vi "CVT_FGV.vi"(0 "command":enum16{"set", "get", "reset", "get all"}(ring), 5 "variable":string, 7 "value in":string, 9 "compressed":bool, 11 "error in":errorcluster) -> (4 "value out":string, 6 "all out":variant, 15 "error out":errorcluster)   [LabVIEW 2011]
panel:
  out "uncompressed":variant
  out "compressed":variant
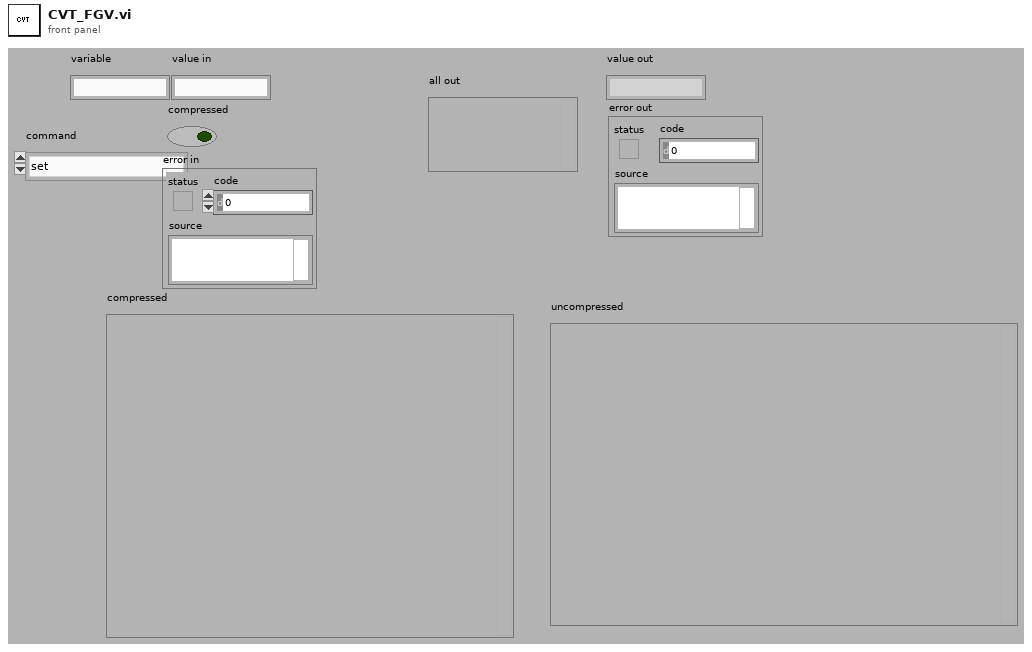
[diagram p1: front panel]
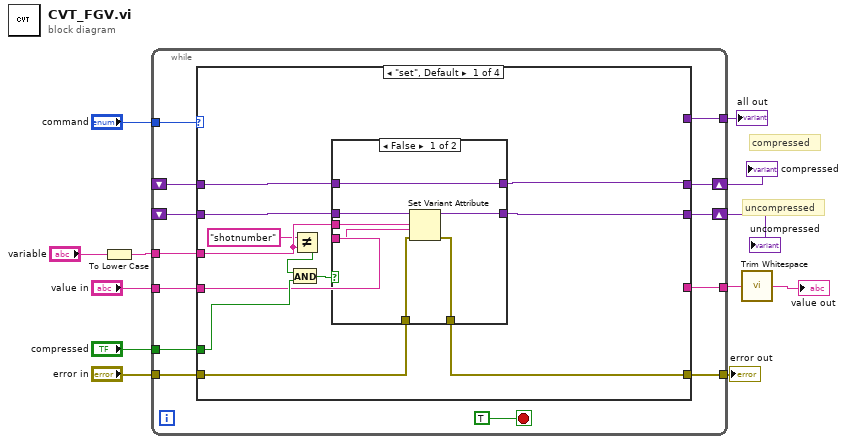
[diagram p0: block diagram]
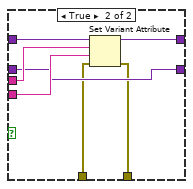
[diagram p2: hidden frame]
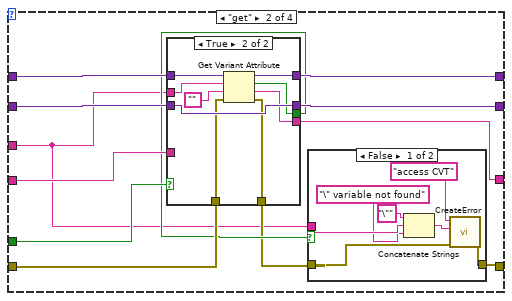
[diagram p3: hidden frame]
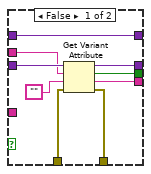
[diagram p5: hidden frame]
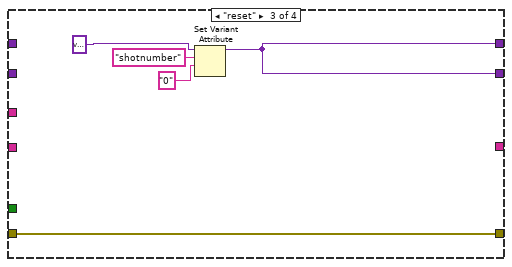
[diagram p6: hidden frame]
diagram:
  # "uncompressed"
  # "compressed"
  n1 = To Lower Case(string="variable") -> (all lower case string=w1:string)
  n2 = while {
    shift-right: [w22] -> w5
    shift-left: _ -> [w23]
    tunnel: "command" -> [w24]
    tunnel: w1 -> [w21]
    tunnel: "value in" -> [w20]
    shift-right: [w18] -> w4
    shift-left: _ -> [w17]
    tunnel: "compressed" -> [w19]
    tunnel: [w16] -> w7
    tunnel: "error in" -> [w15]
    tunnel: [w14] -> w8
    tunnel: [w13] -> w3
    stop <- TRUE stop-if-true
    n3 = case shown="\"set\", Default" w24 {
      tunnel: w23 -> [w37 w62 _ w97]
      tunnel: [w32 w61 w90 w97] -> w22
      tunnel: w21 -> [w31 w52 _ _]
      tunnel: w20 -> [w26 w58 _ _]
      tunnel: w19 -> [w28 w63 _ w98]
      tunnel: [w36 w59 w90 w96] -> w18
      tunnel: w17 -> [w35 w60 _ w96]
      tunnel: [_ w57 _ _] -> w16
      tunnel: w15 -> [w34 w56 w94 w99]
      tunnel: [w33 w53 w94 w99] -> w14
      tunnel: [_ _ _ w95] -> w13
      frame "set", Default {
        n4 = Not Equal?(x="shotnumber", y=w31) -> (x != y?=w29:bool)
        n5 = And(x=w29, y=w28) -> (x .and. y?=w27:bool)
        n6 = case shown="False" w27 {
          tunnel: w37 -> [w40 w51]
          tunnel: [w40 w50] -> w32
          tunnel: w31 -> [w42 w49]
          tunnel: w26 -> [w41 w48]
          tunnel: [w44 w47] -> w36
          tunnel: w35 -> [w43 w47]
          tunnel: w34 -> [w39 w46]
          tunnel: [w38 w45] -> w33
          frame False {
            n7 = Set Variant Attribute(Variant=w43, name=w42, value=w41, error in=w39) -> (Variant out=w44:variant, error out=w38:errorcluster)  [unwired: 1 out]
          }
          frame True {
            n8 = Set Variant Attribute(Variant=w51, name=w49, value=w48, error in=w46) -> (Variant out=w50:variant, error out=w45:errorcluster)  [unwired: 1 out]
          }
        }
      }
      frame "get" {
        n9 = case shown="True" w63 {
          tunnel: w62 -> [w78 w89]
          tunnel: [w78 w88] -> w61
          tunnel: w60 -> [w80 w87]
          tunnel: [w79 w87] -> w59
          tunnel: w52 -> [w77 w86]
          tunnel: w58 -> [_ _]
          tunnel: [w75 w84] -> w57
          tunnel: w56 -> [w74 w83]
          tunnel: [w73 w82] -> w54
          tunnel: [w72 w81] -> w55
          frame False {
            n10 = Get Variant Attribute(Variant=w80, name=w77, default value (empty Variant)="", error in=w74) -> (duplicate Variant=w79:variant, found=w72:bool, value=w75:string, error out=w73:errorcluster)
          }
          frame True {
            n11 = Get Variant Attribute(Variant=w89, name=w86, default value (empty Variant)="", error in=w83) -> (duplicate Variant=w88:variant, found=w81:bool, value=w84:string, error out=w82:errorcluster)
          }
        }
        n12 = case shown="False" w55 {
          tunnel: w54 -> [w70 w71]
          tunnel: [w69 w71] -> w53
          tunnel: w52 -> [w66 _]
          frame False {
            n13 = Concatenate Strings("\"" ("string"), w66, "\" variable not found" ("error message (\"\")")) -> (w65:string)
            n14 = call "CreateError.vi"("user error in"=w70, "error message (\"\")"=w65, "command"="access CVT") -> ("user error  out"=w69:errorcluster)  [unwired: 8 in]
          }
          frame True {
          }
        }
      }
      frame "reset" {
        n15 = Set Variant Attribute(Variant=variant, name="shotnumber", value="0" ("name")) -> (Variant out=w90:variant)  [unwired: 1 in, 2 out]
      }
      frame "get all" {
        n16 = case shown="True" w98 {
          tunnel: w97 -> [_ w101]
          tunnel: w96 -> [w100 _]
          tunnel: [w100 w101] -> w95
          frame False {
          }
          frame True {
          }
        }
      }
    }
  }
  "error out" <- w8
  "compressed" <- w5
  "uncompressed" <- w4
  "all out" <- w3
  n17 = call "Trim Whitespace.vi"("string"=w7) -> ("trimmed string"=→"value out":string)  [unwired: 1 in]
